vi "Write Voltage Schedule.vi"(8 "error in (no error)":errorcluster, 10 "Schedule":u16(ring) items=["Constant", "Ramp", "Function", "Formula"], 11 "ObjectSettings in":refnum<class "ObjectSettings.lvclass">) -> (0 "error out":errorcluster, 3 "ObjectSettings out":refnum<class "ObjectSettings.lvclass">)   [LabVIEW 2019, in "ObjectSettings.lvclass"]
uses:
  ObjectSettings.lvclass
  ObjectSettings.lvclass/ObjectSettings.ctl
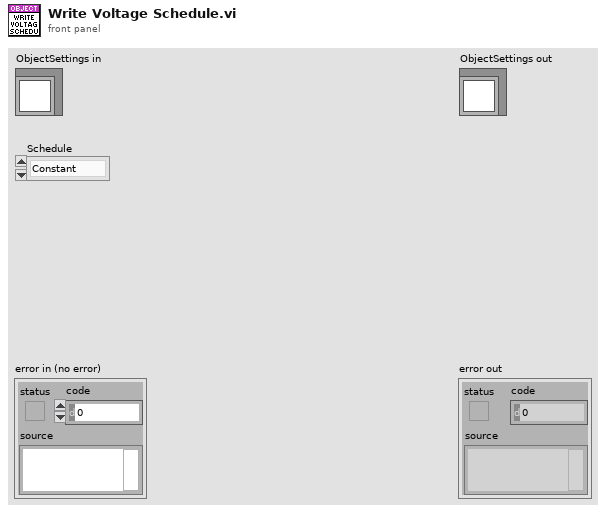
[diagram p1: front panel]
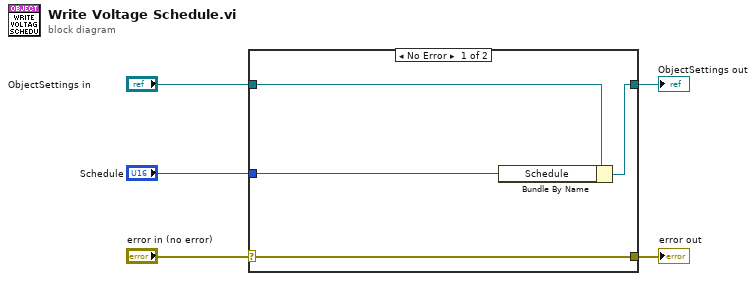
[diagram p0: block diagram]
diagram:
  n1 = case shown="No Error" "error in (no error)" {
    selector: "error in (no error)" -> [w9 w10]
    tunnel: [w9 w10] -> w4
    tunnel: [w7 w11] -> w2
    tunnel: "ObjectSettings in" -> [w8 w11]
    tunnel: "Schedule" -> [w6 _]
    frame No Error {
      n2 = Bundle By Name(cluster=w8, "Schedule"=w6) -> (w7:refnum<class "ObjectSettings.lvclass">)
    }
    frame Error {
    }
  }
  "error out" <- w4
  "ObjectSettings out" <- w2
